vi "LS_372_read_heater_range.vi"(3 "Error In":errorcluster, 5 "VISA (in)":refnum<visa-resource-name>) -> (0 "Error Out":errorcluster, 1 "Numeric":dbl, 2 "VISA (out)":refnum<visa-resource-name>)   [LabVIEW 2018]
panel:
  out "String":string
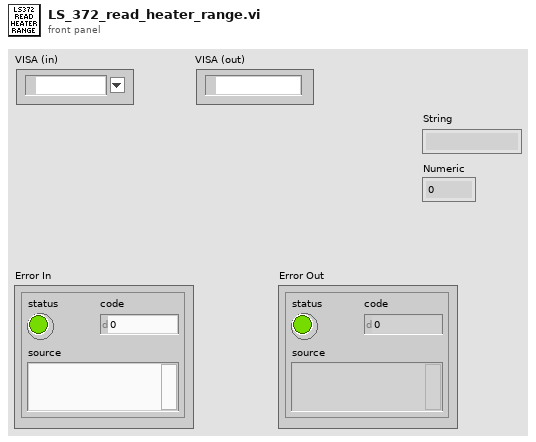
[diagram p1: front panel]
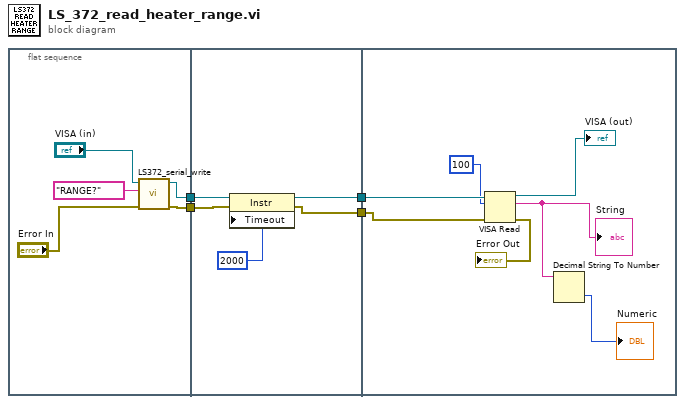
[diagram p0: block diagram]
diagram:
  n1 = flat-sequence {
    tunnel: [w8] -> w4
    tunnel: [w7] -> w3
    tunnel: w4 -> [w14]
    tunnel: w3 -> [w12]
    tunnel: [w13] -> w2
    tunnel: [w11] -> w1
    tunnel: w2 -> [w21]
    tunnel: w1 -> [w19]
    frame #0 {
      n2 = call "LS372_serial_write.vi"("error in (no error)"="Error In", "Write Buffer (\"\")"="RANGE?", "VISA resource name"="VISA (in)") -> ("error out"=w7:errorcluster, "VISA resource name out"=w8:refnum<visa-resource-name>)  [unwired: 6 in, 1 out]
    }
    frame #1 {
      n3 = property class="Instr"(reference=w14, error in=w12, "Timeout"=2000) -> (reference out=w13:refnum<visa-resource-name>, error out=w11:errorcluster)
    }
    frame #2 {
      n4 = VISA Read(VISA resource name=w21, byte count=100, error in (no error)=w19) -> (VISA resource name out=→"VISA (out)":refnum<visa-resource-name>, read buffer=w16:string, error out=→"Error Out":errorcluster)  [unwired: 1 out]
      "String" <- w16
      n5 = Decimal String To Number(string=w16) -> (number=→"Numeric":i32)  [unwired: 2 in, 1 out]
    }
  }
